vi "Format AO DAQ Configuration Log.vi"(8 "error in (no error)":errorcluster, 11 "Instrument.Lockin in":refnum<class "Instrument.Lockin.lvclass">) -> (0 "error out":errorcluster, 2 "Array":T1[](array[typedef]), 3 "Instrument.Lockin out":refnum<class "Instrument.Lockin.lvclass">)   [LabVIEW 2019, in "Instrument.Lockin.lvlib" / "Instrument.Lockin.lvclass"]
uses:
  Instrument.Lockin.lvclass
  Typedefs/Lockin.LogConfiguration.DAQ--Cluster.ctl
  Instrument.Lockin.lvclass/Instrument.Lockin.ctl
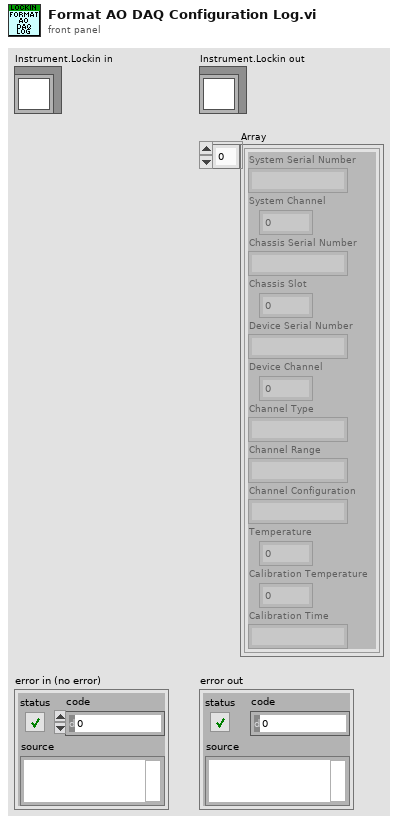
[diagram p1: front panel]
types:
  T1 = typedef "Instrument.Lockin.lvlib/Instrument.Lockin.lvclass/Lockin.LogConfiguration.DAQ--Cluster.ctl" = cluster{"System Serial Number":string, "System Channel":i32, "Chassis Serial Number":string, "Chassis Slot":i32, "Device Serial Number":string, "Device Channel":i32, "Channel Type":string, "Channel Range":string, "Channel Configuration":string, "Temperature":dbl, "Calibration Temperature":dbl, "Calibration Time":string}
  T2 = typedef "Instrument.Lockin.lvlib/Instrument.DAQ.lvclass/AO.Channel--Cluster--Array.ctl" = T3[]
  T3 = typedef "Instrument.Lockin.lvlib/Instrument.DAQ.lvclass/AO.Channel--Cluster.ctl" = cluster{"Enable?":bool, "Channel":i32, "Amplitude":dbl, "Offset":dbl, "Frequency":dbl, "Phase":dbl, "Function":T4, "Sweeping?":bool, "Limit AC":bool, "Limit DC?":bool, "Duty Cycle":bool}
  T4 = typedef "Instrument.Lockin.lvlib/Instrument.DAQ.lvclass/AO.Channel.Function--Enum.ctl" = enum16{"sine", "square", "triangle", "saw"}
  T5 = typedef "Instrument.Lockin.lvlib/Instrument.DAQ.lvclass/DeviceInfo--Cluster.ctl" = cluster{"DeviceName":string, "DevIsSimulated":bool, "DeviceSerialNumber":string, "ProductType":string, "ProductCategory":i32, "ProductNumber":u32, "ChassisNumber":u32, "SlotNumber":u32, "ChassisName":string, "ChassisSerialNumber":string, "DevTemp":dbl, "SelfCal.LastDate/Time":string, "SelfCal.LastTemp":dbl, "calibration due?":bool}
  T6 = typedef "Instrument.Lockin.lvlib/Instrument.DAQ.lvclass/DAQ.Config.AO--Cluster--Array.ctl" = cluster{"Channels":tag, "Range":T7, "terminal configuration":T8, "Type":T9}[]
  T7 = typedef "Instrument.Lockin.lvlib/Instrument.DAQ.lvclass/DAQ.Config.AO.Range--enum.ctl" = enum16{"±0.1", "±1.0", "±10.0", ""}
  T8 = typedef "Instrument.Lockin.lvlib/Instrument.DAQ.lvclass/DAQ.TerminalConfiguration--ring.ctl" = i32
  T9 = typedef "Instrument.Lockin.lvlib/Instrument.DAQ.lvclass/DAQ.Type--enum.ctl" = enum16{"None", "USB-4431", "PXI-446x"}
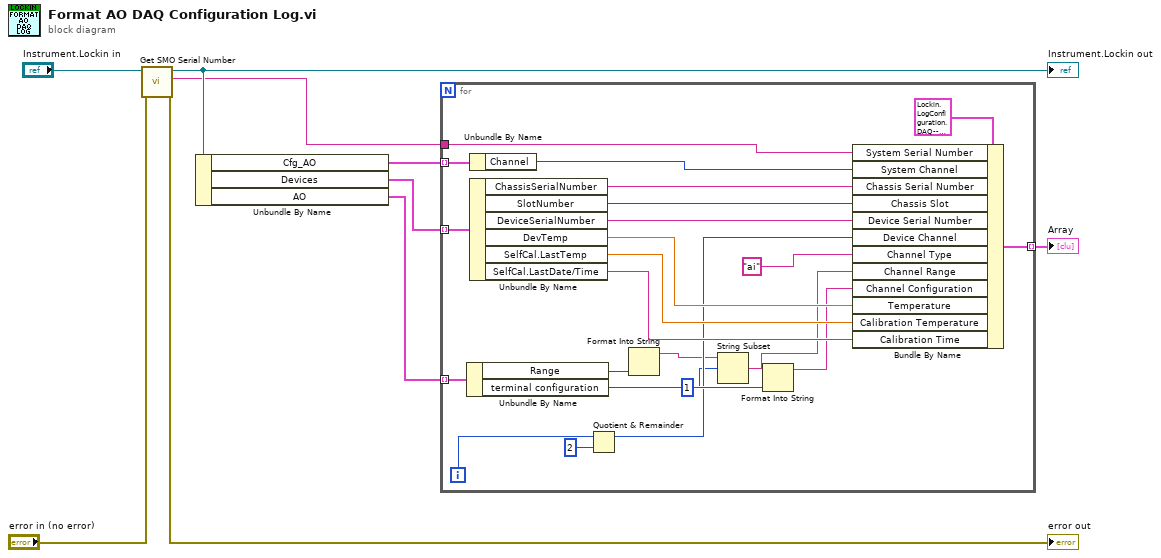
[diagram p0: block diagram]
diagram:
  n1 = call-dynamic "Get SMO Serial Number.vi"("error in (no error)"="error in (no error)", "Instrument.Lockin in"="Instrument.Lockin in") -> ("error out"=→"error out":errorcluster, "Serial Number"=w7:string, "Instrument.Lockin out"=w9:refnum<class "Instrument.Lockin.lvclass">)  [unwired: 7 in]
  "Instrument.Lockin out" <- w9
  n2 = Unbundle By Name(w9) -> ("Cfg_AO"=w4:T2, "Devices"=w5:T5[], "AO"=w6:T6)
  n3 = for {
    tunnel: [w32] -> w2 mode=indexing
    tunnel: w7 -> [w16]
    tunnel: w5 -> [w30] mode=indexing
    tunnel: w4 -> [w29] mode=indexing
    tunnel: w6 -> [w21] mode=indexing
    i -> [w15]
    n4 = Unbundle By Name(w21) -> ("Range"=w20:T7, "terminal configuration"=w18:T8)
    n5 = Unbundle By Name(w29) -> ("Channel"=w28:i32)
    n6 = Unbundle By Name(w30) -> ("ChassisSerialNumber"=w27:string, "SlotNumber"=w26:u32, "DeviceSerialNumber"=w25:string, "DevTemp"=w22:dbl, "SelfCal.LastTemp"=w23:dbl, "SelfCal.LastDate/Time"=w24:string)
    n7 = Quotient & Remainder(x=w15, y=2) -> (x-y*floor(x/y)=w13:i32)  [unwired: 1 out]
    n8 = Format Into String(w20) -> (resulting string=w11:string)  [unwired: 3 in, 1 out]
    n9 = String Subset(string=w11, offset (0)=1) -> (substring=w10:string)  [unwired: 1 in]
    n10 = Format Into String(w18) -> (resulting string=w19:string)  [unwired: 3 in, 1 out]
    n11 = Bundle By Name(cluster=T1 {"System Serial Number"="", "System Channel"=0, "Chassis Serial Number"="", "Chassis Slot"=0, "Device Serial Number"="", "Device Channel"=0, "Channel Type"="", "Channel Range"="", "Channel Configuration"="", "Temperature"=0.0, "Calibration Temperature"=0.0, "Calibration Time"=""} ("DAQ Configuration"), "System Serial Number"=w16, "System Channel"=w28, "Chassis Serial Number"=w27, "Chassis Slot"=w26, "Device Serial Number"=w25, "Device Channel"=w13, "Channel Type"="ai" ("format string"), "Channel Range"=w10, "Channel Configuration"=w19, "Temperature"=w22, "Calibration Temperature"=w23, "Calibration Time"=w24) -> (w32:T1)
  }
  "Array" <- w2
